vi "cRIO Backplane Info.vi"(8 "error in (no error)":errorcluster, 11 "session in":refnum<k21>="localhost") -> (0 "error out":errorcluster, 1 "Number of Slots":i32[](array[numeric]), 2 "Chasses Info":T1[](array[typedef]))   [LabVIEW 2017, in "cRIODetectHW.lvlib"]
doc: "Gets information about the chassis used in the specified session, such as model name, model code, and serial number."
uses:
  <vilib>/addons/cRIODetectHW/cRIODetectHW.lvlib
  <vilib>/addons/cRIODetectHW/control/cRIO Product Info.ctl
  <vilib>/nisyscfg/Initialize (Control).vi
  <vilib>/nisyscfg/Find Hardware.vi
  <vilib>/nisyscfg/Close (Hardware).vi
  <vilib>/nisyscfg/Close (Filter).vi
  <resource>/objmgr/nicriosae.rc
  <resource>/objmgr/niflexriosae.rc
  <vilib>/nisyscfg/nisyscfg.lvlib
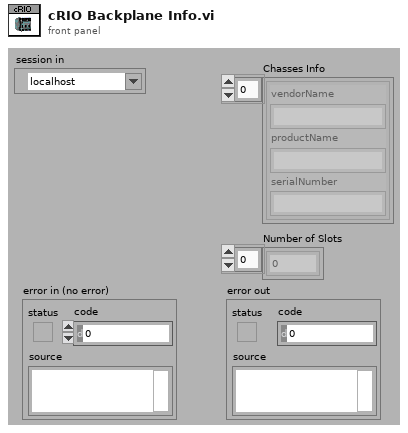
[diagram p1: front panel]
types:
  T1 = typedef "cRIODetectHW.lvlib/cRIO Product Info.ctl" = cluster{"vendorName":string, "productName":string, "serialNumber":string}
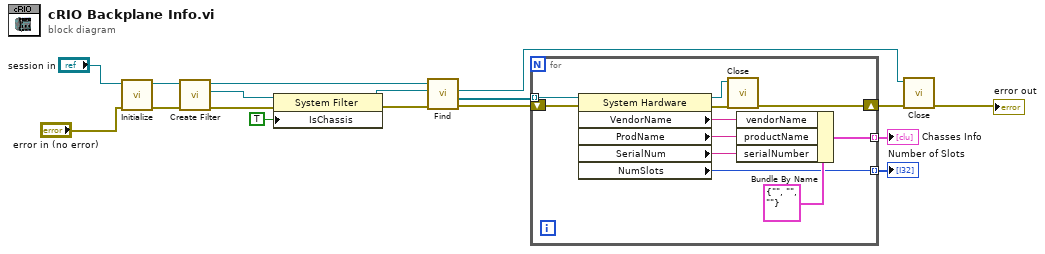
[diagram p0: block diagram]
diagram:
  n1 = call-poly <vilib>:"Initialize.vi"("error in (no error)"="error in (no error)", "Target (localhost)"="session in") -> ("error out"=w4:errorcluster, "Session out"=w5:refnum<k21>)  [unwired: 7 in, 1 out]
  n2 = call <vilib>:"Create Filter.vi"("error in (no error)"=w4, "Session in"=w5) -> ("error out"=w16:errorcluster, "Filter out"=w17:refnum<k20>, "Session out"=w14:refnum<k21>)  [unwired: 7 in]
  n3 = property class="System Filter"(reference=w17, error in=w16, "IsChassis"=TRUE ("Is Chassis")) -> (reference out=w13:refnum<k20>, error out=w12:errorcluster)
  n4 = call-poly <vilib>:"Find.vi"("error in (no error)"=w12, "Filter in"=w13, "Session in"=w14) -> ("error out"=w11:errorcluster, "Resources out"=w10:refnum<k20>[], "Filter out"=w8:refnum<k20>)  [unwired: 5 in, 1 out]
  n5 = for {
    tunnel: w10 -> [w28] mode=indexing
    shift-right: [w25] -> w9
    shift-left: w11 -> [w24]
    tunnel: [w21] -> w3 mode=indexing
    tunnel: [w18] -> w1 mode=indexing
    n6 = property class="System Hardware"(reference=w28, error in=w24) -> (reference out=w26:refnum<k20>, error out=w27:errorcluster, "VendorName"=w23:string, "ProdName"=w20:string, "SerialNum"=w19:string, "NumSlots"=w18:i32)
    n7 = call-poly <vilib>:"Close.vi"("error in (no error)"=w27, "Resource in"=w26) -> ("error out"=w25:errorcluster)  [unwired: 9 in]
    n8 = Bundle By Name(cluster=T1 {"vendorName"="", "productName"="", "serialNumber"=""} ("cRIO Backplane Info"), "vendorName"=w23, "productName"=w20, "serialNumber"=w19) -> (w21:T1)
  }
  "Chasses Info" <- w3
  "Number of Slots" <- w1
  n9 = call-poly <vilib>:"Close.vi"("error in (no error)"=w9, "Filter in"=w8) -> ("error out"=→"error out":errorcluster)  [unwired: 9 in]
